vi "PathPlanner_GridPosition_HashCode.vi"(11 "GridPosition":T1) -> (3 "HashCode":i32)   [LabVIEW 2019, in "PathPlanner24.lvlib"]
uses:
  PathPlanner24.lvlib
  TypeDef/PathPlannerFinderGridPosition.ctl
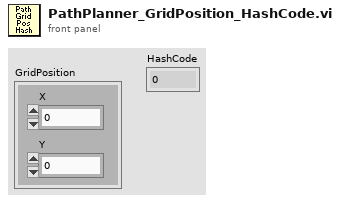
[diagram p1: front panel]
types:
  T1 = typedef "PathPlanner24.lvlib/PathPlannerFinderGridPosition.ctl" = cluster{"X":i32, "Y":i32}
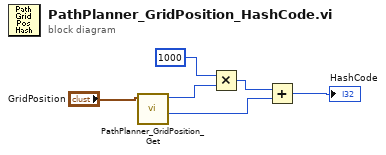
[diagram p0: block diagram]
diagram:
  n1 = call "PathPlanner_GridPosition_Get.vi"("GridPosition"="GridPosition") -> ("Int Y"=w3:i32, "Int X"=w5:i32)  [unwired: 9 in]
  n2 = Multiply(x=1000, y=w5) -> (x*y=w4:i32)
  n3 = Add(x=w4, y=w3) -> (x+y=→"HashCode":i32)
